vi "Config TDMS File for Asynchronous Read.vi"(0 "TDMS read controls array":T1[](array[typedef]), 1 "max asynchronous reads":u32=8, 2 "Samples per Write":u32=1024000 format="%.3p", 3 "chunks":u32=16 caption="Chuncks" format="%.0p", 5 "HSS refnum in":refnum<k20>, 7 "disable buffering? (T)":bool=TRUE, 9 "tx config":T2={"rf enable 0"=FALSE, "rf config 0"={"antenna"="TX1", "frequency"=2000000000.0, "lo frequency"=-1.0, "level"=0.0}, "rf enable 1"=FALSE, "rf config 1"={"antenna"="TX1", "frequency"=2000000000.0, "lo frequency"=-1.0, "level"=0.0}, "transfer mode"=enum."Finite", "sample rate"=10000000.0, "start trigger"=enum."Immediate"} {"sample rate" format="%#.3pS/s"; "rf config 0"."level" format="%#_gdBm"; "rf config 0"."lo frequency" format="%#.3pHz"; "rf config 0"."frequency" format="%#.3pHz"; "rf config 1"."level" format="%#_gdBm"; "rf config 1"."lo frequency" format="%#.3pHz"; "rf config 1"."frequency" format="%#.3pHz"}, 11 "error in (no error)":errorcluster, 12 "Queue in":refnum<queue>, 13 "Infinite Generation":bool) -> (4 "TDMS read control array out":T1[](array[typedef]), 6 "channels up?":bool[](array[boolean]), 8 "read process finished?":bool, 15 "error out":errorcluster)   [LabVIEW 2018]
doc: "Configure TDMS Settings for asynchronous write"
uses:
  TypeDefs/Tx Config.ctl
  2954/SubVIs/Start Trigger.ctl
  TypeDefs/TDMS read.ctl
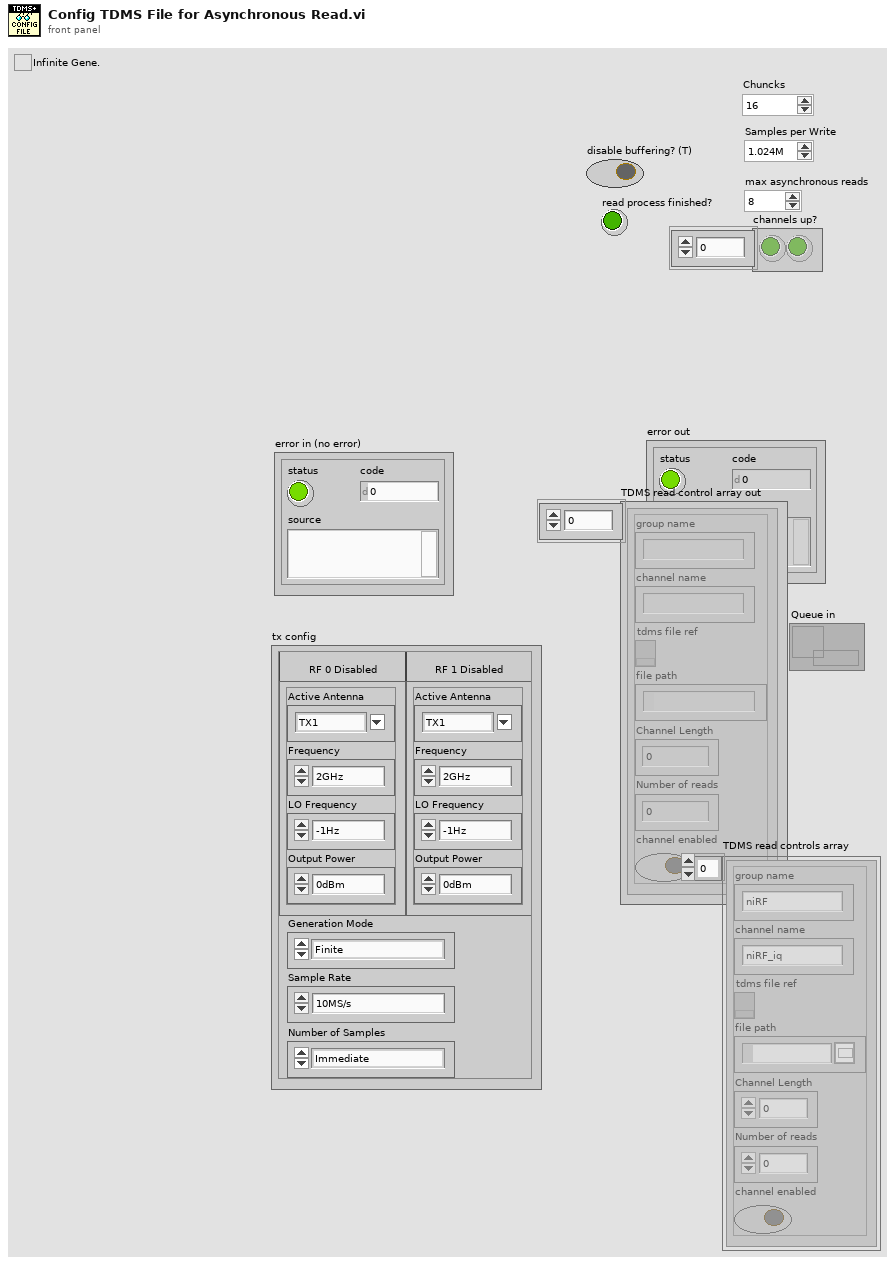
[diagram p1: front panel]
types:
  T1 = typedef "TDMS read.ctl" = cluster{"group name":string, "channel name":string, "tdms file ref":refnum<k34>, "file path":path, "Channel Length":i64, "Number of reads":i64, "channel enabled":bool}
  T2 = typedef "Tx Config.ctl" = cluster{"rf enable 0":bool, "rf config 0":cluster{"antenna":string, "frequency":dbl, "lo frequency":dbl, "level":dbl}, "rf enable 1":bool, "rf config 1":cluster{"antenna":string, "frequency":dbl, "lo frequency":dbl, "level":dbl}, "transfer mode":enum16{"Finite", "Continuous"}, "sample rate":dbl, "start trigger":T3}
  T3 = typedef "Start Trigger.ctl" = enum8{"Software", "Digital Edge", "Rx Start Trigger", "Tx Start Trigger", "Immediate", "Future Time Event"}
  T4 = enum16{"open", "open or create", "create or replace", "create", "open (read-only)"}
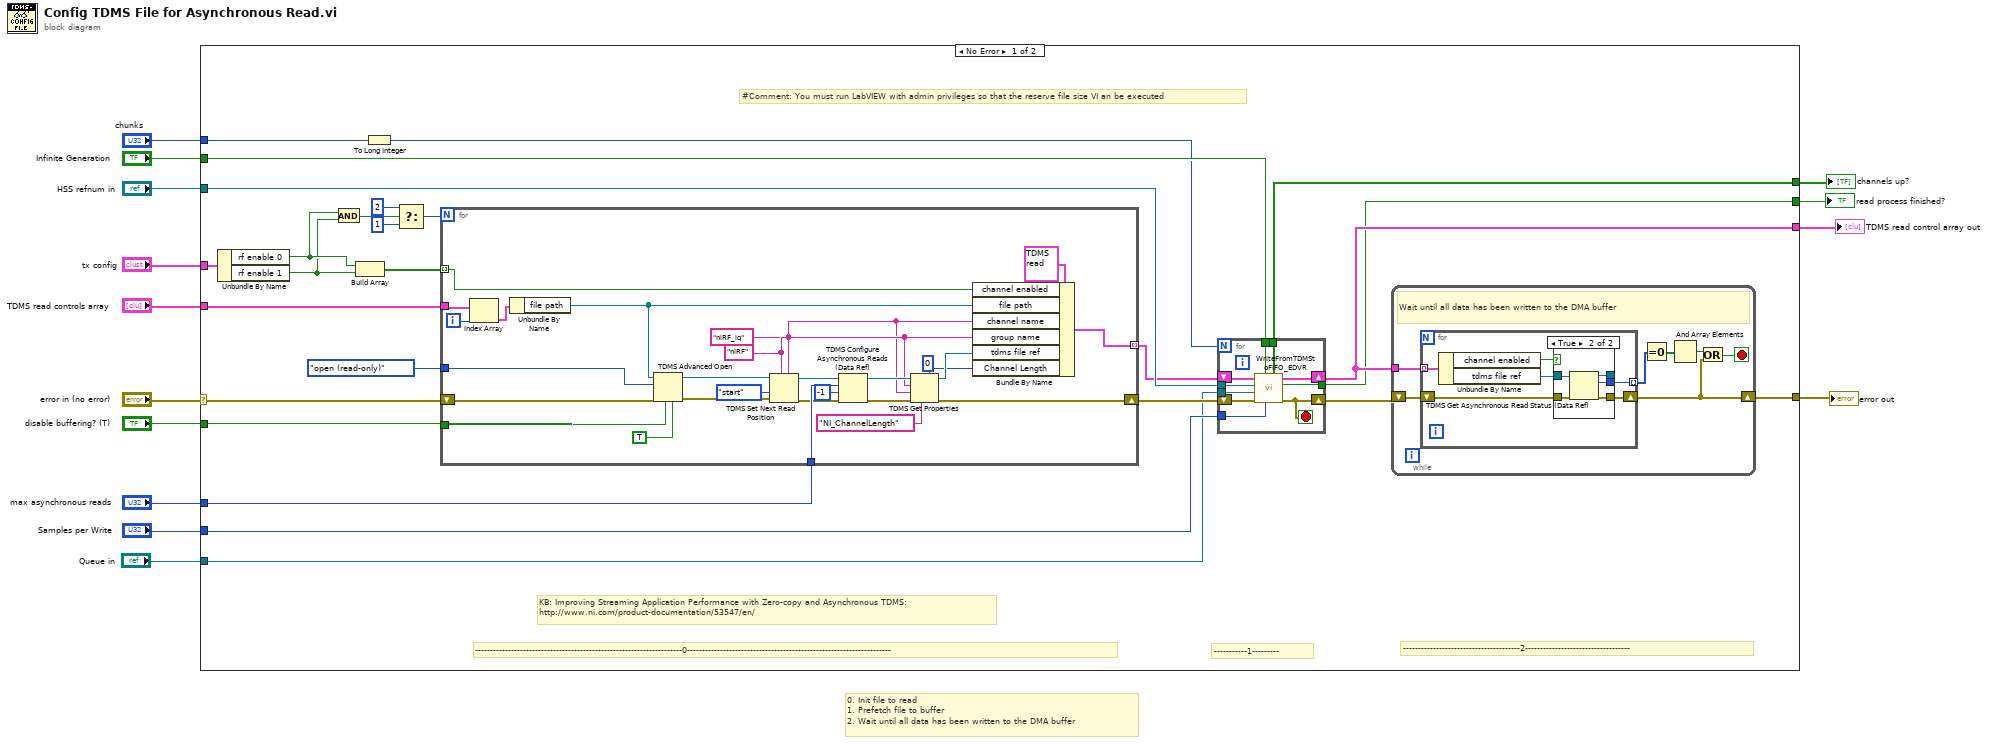
[diagram p0: block diagram]
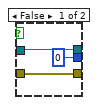
[diagram p2: hidden frame]
diagram:
  # "0. Init file to read\n1. Prefetch file to buffer\n2. Wait until all data has been written to the DMA buffer"
  n1 = case shown="No Error" "error in (no error)" {
    selector: "error in (no error)" -> [w29 w99]
    tunnel: "chunks" -> [w40 _]
    tunnel: [w38 w99] -> w13
    tunnel: "max asynchronous reads" -> [w36 _]
    tunnel: "disable buffering? (T)" -> [w35 _]
    tunnel: "Samples per Write" -> [w23 _]
    tunnel: [w34 _] -> w9
    tunnel: "tx config" -> [w33 _]
    tunnel: "HSS refnum in" -> [w31 _]
    tunnel: "Infinite Generation" -> [w26 _]
    tunnel: [w25 _] -> w5
    tunnel: [w28 _] -> w3
    tunnel: "TDMS read controls array" -> [w27 _]
    tunnel: "Queue in" -> [w22 _]
    frame No Error {
      # "---------------------------------------2-----------------------------------"
      # "-----------1---------"
      # "---------------------------------------------------------------------0--------------------------------------------------------------------"
      # "KB: Improving Streaming Application Performance with Zero-copy and Asynchronous TDMS:\nhttp://www.ni.com/product-documentation/53547/en/"
      # "#Comment: You must run LabVIEW with admin privileges so that the reserve file size VI an be executed"
      n2 = Unbundle By Name(w33) -> ("rf enable 0"=w17:bool, "rf enable 1"=w16:bool)
      n3 = And(x=w17, y=w16) -> (x .and. y?=w21:bool)
      n4 = Build Array(w17, w16) -> (w15:bool[])
      n5 = To Long Integer(number=w40) -> (32bit integer=w24:i32)
      n6 = Select(t=2, s=w21, f=1) -> (s? t:f=w18:i32)
      n7 = for {
        N: w18 -> [_]
        shift-right: [w98] -> w32
        shift-left: w29 -> [w94]
        tunnel: T4."open (read-only)" ("operation (0:open)") -> [w97]
        tunnel: w36 -> [w96]
        tunnel: w35 -> [w95]
        tunnel: [w93] -> w30 mode=indexing
        tunnel: w27 -> [w91]
        tunnel: w15 -> [w72] mode=indexing
        i -> [w89]
        w76 = "niRF_iq" ("group name")
        w77 = "niRF" ("group name")
        n8 = Index Array(array=w91, index=w89) -> (element=w90:T1)
        n9 = Unbundle By Name(w90) -> ("file path"=w92:path)
        n10 = TDMS Advanced Open(4:TRUE ("enable asynchronous? (T)"), 6:w95, 8:w94, 10:w97, 11:w92) -> (0:w82:errorcluster, 3:w83:refnum<k34>)  [unwired: 1 out]
        n11 = TDMS Set Next Read Position(5:w76, 7:w77, 8:w82, 9:enum16{"start", "end"}."start" ("from (0: start)"), 11:w83) -> (0:w86:errorcluster, 3:w85:refnum<k34>)  [unwired: 1 in]
        n12 = TDMS Configure Asynchronous Reads (Data Ref)(8:w86, 9:i64 -1 ("total size (in bytes) (-1)"), 10:w96, 11:w85) -> (0:w78:errorcluster, 3:w80:refnum<k34>)  [unwired: 1 in]
        n13 = TDMS Get Properties(5:i64 0 ("total size (in bytes) (-1)"), 7:"NI_ChannelLength" ("property name"), 8:w78, 9:w76, 10:w77, 11:w80) -> (0:w98:errorcluster, 3:w79:refnum<k34>, 4:w73:i64)  [unwired: 3 out]
        n14 = Bundle By Name(cluster=T1 {"group name"="niRF", "channel name"="niRF_iq", "tdms file ref"=refnum, "file path"=path "", "Channel Length"=0, "Number of reads"=0, "channel enabled"=FALSE} ("input cluster"), "channel enabled"=w72, "file path"=w92, "channel name"=w76, "group name"=w77, "tdms file ref"=w79, "Channel Length"=w73) -> (w93:T1)
      }
      n15 = for {
        N: w24 -> [_]
        tunnel: w23 -> [w43]
        tunnel: [w50] -> w34
        tunnel: w31 -> [w48]
        shift-right: [w42] -> w39
        shift-left: w32 -> [w49]
        tunnel: w26 -> [w45]
        tunnel: [w44] -> w25
        shift-right: [w46] -> w28
        shift-left: w30 -> [w47]
        tunnel: w22 -> [w41]
        stop <- w42 stop-if-true
        n16 = call "WriteFromTDMStoFIFO_EDVR.vi"("Samples per Write"=w43, "Infinite Generation"=w45, "error in (no error)"=w49, "Queue in"=w41, "HSS refnum in"=w48, "TDMS read controls in"=w47) -> ("error out"=w42:errorcluster, "read process finished?"=w44:bool, "TDMS read controls out"=w46:T1[], "Channels Running?"=w50:bool[])  [unwired: 2 in]
      }
      n17 = while {
        shift-right: [w54] -> w38
        shift-left: w39 -> [w57]
        tunnel: w28 -> [w51]
        stop <- w55 stop-if-true
        # "Wait until all data has been written to the DMA buffer"
        n18 = for {
          tunnel: [w62] -> w56 mode=indexing
          shift-right: [w61] -> w54
          shift-left: w57 -> [w63]
          tunnel: w51 -> [w60] mode=indexing
          n19 = Unbundle By Name(w60) -> ("channel enabled"=w58:bool, "tdms file ref"=w59:refnum<k34>)
          n20 = case shown="True" w58 {
            tunnel: w63 -> [w65 w71]
            tunnel: [u32 0 ("number of pending reads") w70] -> w62
            tunnel: [w66 w69] -> _
            tunnel: [w65 w68] -> w61
            tunnel: w59 -> [w66 w67]
            frame False {
            }
            frame True {
              n21 = TDMS Get Asynchronous Read Status (Data Ref)(8:w71, 11:w67) -> (0:w68:errorcluster, 2:w70:u32, 3:w69:refnum<k34>)
            }
          }
        }
        n22 = Equal To 0?(x=w56) -> (x = 0?=w53:bool[])
        n23 = And Array Elements(Boolean array=w53) -> (logical AND=w52:bool)
        n24 = Or(x=w52, y=w54) -> (x .or. y?=w55:bool)
      }
    }
    frame Error {
    }
  }
  "error out" <- w13
  "read process finished?" <- w5
  "channels up?" <- w9
  "TDMS read control array out" <- w3
